vi "Cycle.vi"(8 "error in (no error)":errorcluster, 11 "MouseBar In":refnum<class "MouseBar.lvclass">) -> (0 "error out":errorcluster, 3 "MouseBar Out":refnum<class "MouseBar.lvclass">)   [LabVIEW 2011, in "MouseBar.lvclass"]
uses:
  MouseBar.lvclass
  Trial Based Experiment Statechart/PassiveExperiment/PassiveExperiment.lvclass
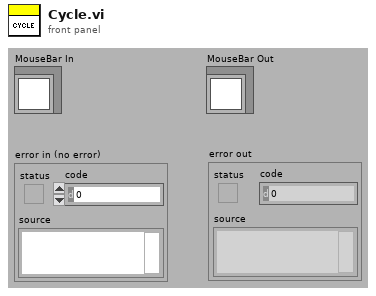
[diagram p1: front panel]
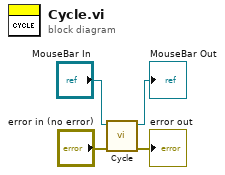
[diagram p0: block diagram]
diagram:
  n1 = call-parent "Cycle.vi"("error in (no error)"="error in (no error)", "PassiveExperiment In"="MouseBar In") -> ("error out"=→"error out":errorcluster, "PassiveExperiment Out"=→"MouseBar Out":refnum<class "MouseBar.lvclass">)  [unwired: 8 in]
